vi "mainWholeBrainImager.vi"   [LabVIEW 2017]
uses:
  globalDevices.vi
  globalUtilities.vi
  <userlib>/Hamamatsu Video Capture/tm_getframe16_40.vi
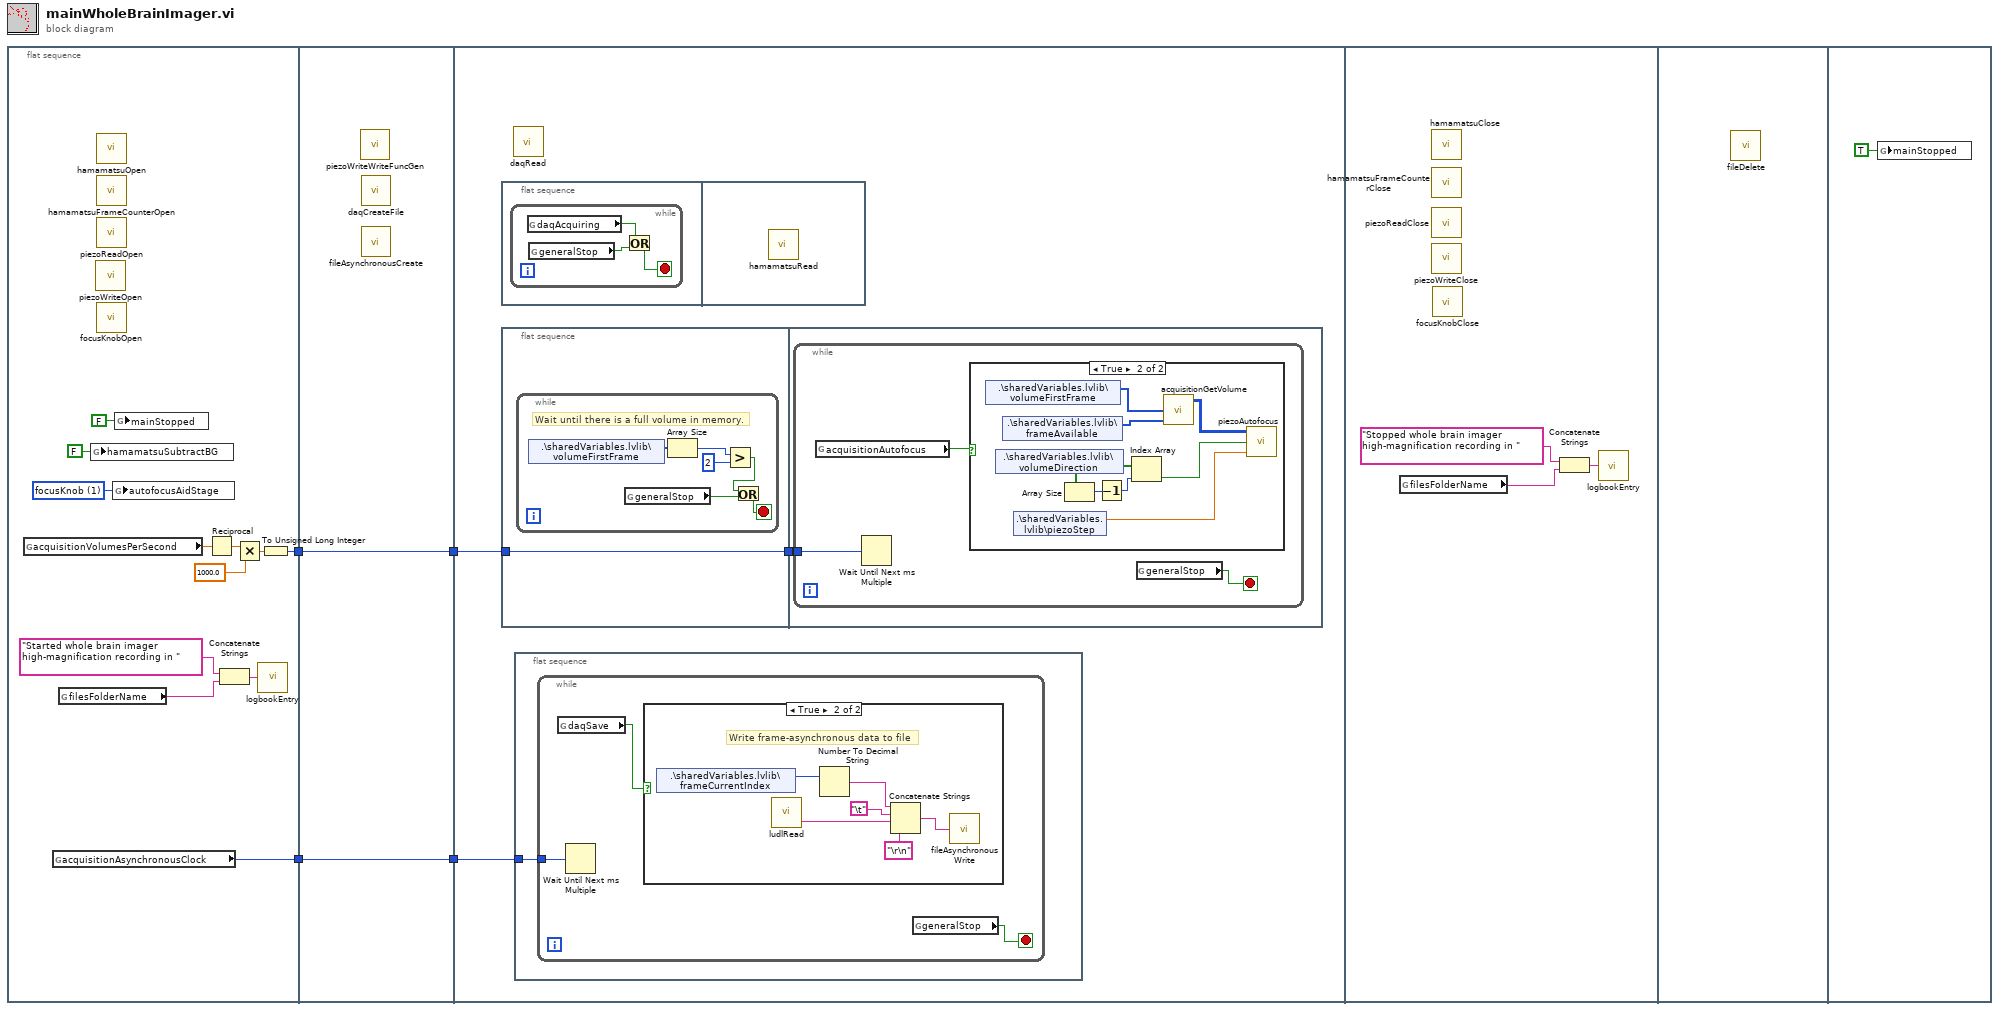
[diagram p0: block diagram]
diagram:
  n1 = flat-sequence {
    tunnel: [w10] -> w4
    tunnel: [w8] -> w1
    tunnel: w4 -> [w18]
    tunnel: [w18] -> w3
    tunnel: [w17] -> w2
    tunnel: w1 -> [w17]
    tunnel: w3 -> [w20]
    tunnel: w2 -> [w19]
    frame #0 {
      w9 = u16 1 items=["none", "focusKnob"] ("autofocusAidStage")
      n2 = global read "globalUtilities.vi" "acquisitionVolumesPerSecond"() -> (w14:dbl)
      n3 = global read "globalUtilities.vi" "acquisitionAsynchronousClock"() -> (w8:u32)
      n4 = global read "globalUtilities.vi" "filesFolderName"() -> (w6:string)
      n5 = global write "globalDevices.vi" "hamamatsuSubtractBG"(FALSE ("hamamatsuSubtractBG")) -> ()
      n6 = call "piezoWriteOpen.vi"() -> ()  [unwired: 2 in]
      n7 = call "hamamatsuOpen.vi"() -> ()  [unwired: 4 out]
      n8 = call "hamamatsuFrameCounterOpen.vi"() -> ()  [unwired: 12 in]
      n9 = call "piezoReadOpen.vi"() -> ()  [unwired: 6 in]
      n10 = call "focusKnobOpen.vi"() -> ()  [unwired: 12 in]
      n11 = global write "globalDevices.vi" "autofocusAidStage"(w9) -> ()
      n12 = global write "globalUtilities.vi" "mainStopped"(FALSE ("mainStopped")) -> ()
      n13 = Reciprocal(x=w14) -> (1/x=w13:dbl)
      n14 = Concatenate Strings("Started whole brain imager high-magnification recording in ", w6) -> (w5:string)
      n15 = Multiply(x=w13, y=1000.0) -> (x*y=w11:dbl)
      n16 = call "logbookEntry.vi"("Log book entry"=w5) -> ()  [unwired: 2 out]
      n17 = To Unsigned Long Integer(number=w11) -> (unsigned 32bit integer=w10:u32)
    }
    frame #1 {
      n18 = call "piezoWriteWriteFuncGen.vi"() -> ()  [unwired: 12 in]
      n19 = call "daqCreateFile.vi"() -> ()  [unwired: 12 in]
      n20 = call "fileAsynchronousCreate.vi"() -> ()  [unwired: 12 in]
    }
    frame #2 {
      n21 = flat-sequence {
        frame #0 {
          n22 = while {
            stop <- w53 stop-if-true
            n23 = global read "globalUtilities.vi" "daqAcquiring"() -> (w52:bool)
            n24 = global read "globalUtilities.vi" "generalStop"() -> (w51:bool)
            n25 = Or(x=w52, y=w51) -> (x .or. y?=w53:bool)
          }
        }
        frame #1 {
          n26 = call "hamamatsuRead.vi"() -> ()  [unwired: 12 in]
        }
      }
      n27 = flat-sequence {
        tunnel: [w32] -> w21
        tunnel: w20 -> [w32]
        tunnel: w21 -> [w39]
        frame #0 {
          n28 = while {
            stop <- w34 stop-if-true
            # "Wait until there is a full volume in memory."
            n29 = shared-variable ".\\sharedVariables.lvlib\\volumeFirstFrame"() -> (w38:u32[])  [unwired: 1 in, 1 out]
            n30 = global read "globalUtilities.vi" "generalStop"() -> (w33:bool)
            n31 = Array Size(array=w38) -> (size(s)=w37:i32)
            n32 = Greater?(x=w37, y=2) -> (0:w35:bool)
            n33 = Or(x=w35, y=w33) -> (x .or. y?=w34:bool)
          }
        }
        frame #1 {
          n34 = while {
            tunnel: w39 -> [w41]
            stop <- w42 stop-if-true
            n35 = global read "globalUtilities.vi" "acquisitionAutofocus"() -> (w40:bool)
            n36 = Wait Until Next ms Multiple(millisecond multiple=w41) -> ()  [unwired: 1 out]
            n37 = case shown="True" w40 {
              frame False {
              }
              frame True {
                n38 = shared-variable ".\\sharedVariables.lvlib\\volumeFirstFrame"() -> (w50:u32[])  [unwired: 1 in, 1 out]
                n39 = shared-variable ".\\sharedVariables.lvlib\\volumeDirection"() -> (w46:bool[])  [unwired: 1 in, 1 out]
                n40 = shared-variable ".\\sharedVariables.lvlib\\frameAvailable"() -> (w49:i32[])  [unwired: 1 in, 1 out]
                n41 = shared-variable ".\\sharedVariables.lvlib\\piezoStep"() -> (w43:dbl)  [unwired: 1 in, 1 out]
                n42 = Array Size(array=w46) -> (size(s)=w47:i32)
                n43 = Decrement(x=w47) -> (x-1=w48:i32)
                n44 = Index Array(array=w46, index=w48) -> (element=w44:bool)
                n45 = call "acquisitionGetVolume.vi"("frameAvailable"=w49, "volumeFirstFrame"=w50) -> ("volume out"=w45:u16[][][])  [unwired: 1 in, 2 out]
                n46 = call "piezoAutofocus.vi"("piezoStep"=w43, "volumeDirection"=w44, "volumeIn"=w45) -> ()  [unwired: 1 out]
              }
            }
            n47 = global read "globalUtilities.vi" "generalStop"() -> (w42:bool)
          }
        }
      }
      n48 = call "daqRead.vi"() -> ()  [unwired: 3 in]
      n49 = flat-sequence {
        tunnel: w19 -> [w22]
        frame #0 {
          n50 = while {
            tunnel: w22 -> [w25]
            stop <- w24 stop-if-true
            n51 = global read "globalUtilities.vi" "daqSave"() -> (w23:bool)
            n52 = Wait Until Next ms Multiple(millisecond multiple=w25) -> ()  [unwired: 1 out]
            n53 = case shown="True" w23 {
              frame False {
              }
              frame True {
                # "Write frame-asynchronous data to file"
                n54 = shared-variable ".\\sharedVariables.lvlib\\frameCurrentIndex"() -> (w29:i32)  [unwired: 1 in, 1 out]
                n55 = call "ludlRead.vi"() -> ("string"=w27:string)  [unwired: 1 in, 2 out]
                n56 = Number To Decimal String(number=w29) -> (decimal integer string=w28:string)  [unwired: 1 in]
                n57 = Concatenate Strings(w28, "\t", w27, "\r\n" ("string")) -> (w31:string)
                n58 = call "fileAsynchronousWrite.vi"("line"=w31) -> ()  [unwired: 1 in]
              }
            }
            n59 = global read "globalUtilities.vi" "generalStop"() -> (w24:bool)
          }
        }
      }
    }
    frame #3 {
      n60 = global read "globalUtilities.vi" "filesFolderName"() -> (w56:string)
      n61 = call "hamamatsuClose.vi"() -> ()  [unwired: 1 out]
      n62 = call "hamamatsuFrameCounterClose.vi"() -> ()  [unwired: 12 in]
      n63 = call "piezoReadClose.vi"() -> ()  [unwired: 1 in]
      n64 = call "piezoWriteClose.vi"() -> ()  [unwired: 1 in]
      n65 = call "focusKnobClose.vi"() -> ()  [unwired: 12 in]
      n66 = Concatenate Strings("Stopped whole brain imager high-magnification recording in ", w56) -> (w55:string)
      n67 = call "logbookEntry.vi"("Log book entry"=w55) -> ()  [unwired: 2 out]
    }
    frame #4 {
      n68 = call "fileDelete.vi"() -> ()  [unwired: 12 in]
    }
    frame #5 {
      n69 = global write "globalUtilities.vi" "mainStopped"(TRUE ("mainStopped")) -> ()
    }
  }
